vi "Validate Alias Values.vi"(8 "error in (no error)":errorcluster, 10 "Endpoint":string, 11 "Alias":string) -> (0 "error out":errorcluster, 1 "Valid":bool)   [LabVIEW 2019, in "Routing and Faulting System Explorer.lvlib"]
uses:
  Routing and Faulting System Explorer.lvlib
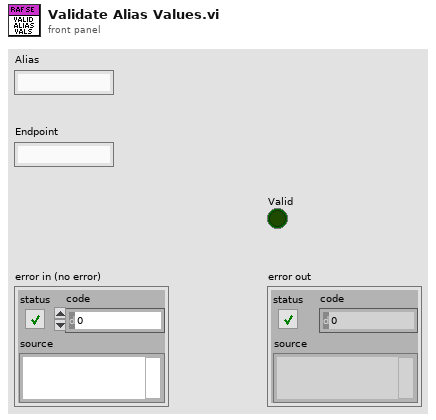
[diagram p1: front panel]
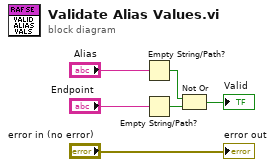
[diagram p0: block diagram]
diagram:
  n1 = Empty String/Path?(string/path="Alias") -> (empty?=w5:bool)
  n2 = Empty String/Path?(string/path="Endpoint") -> (empty?=w6:bool)
  n3 = Not Or(1:w6, 2:w5) -> (0:→"Valid":bool)
  "error out" <- "error in (no error)"
